vi "Translation3d_ToTranslation2d.vi"(11 "In Translation3d":T2 {"Z" format="%14.3f"; "Y" format="%14.3f"; "X" format="%14.3f"}) -> (3 "Translation2d":T1 {"Y" format="%14.3f"; "X" format="%14.3f"})   [LabVIEW 2019, in "Trajectory_Library.lvlib"]
doc: "Returns the X and Ycomponents of the translation.\n\nParameters\n - IN Translation - This Translation data structure\n\nReturns:\n - X- The X component of the translation.\n - Y- The Y component of the translation."
uses:
  TRANSLATION3D.ctl
  Trajectory_Library.lvlib
  TRANSLATION2D.ctl
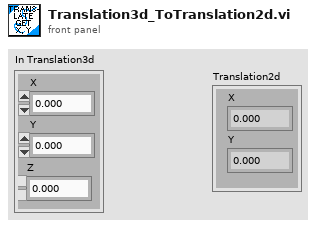
[diagram p1: front panel]
types:
  T1 = typedef "Trajectory_Library.lvlib/TRANSLATION2D.ctl" = cluster{"X":dbl, "Y":dbl}
  T2 = typedef "Trajectory_Library.lvlib/TRANSLATION3D.ctl" = cluster{"X":dbl, "Y":dbl, "Z":dbl}
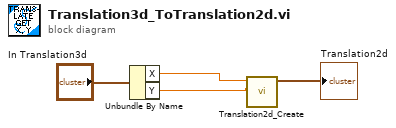
[diagram p0: block diagram]
diagram:
  n1 = Unbundle By Name("In Translation3d") -> ("X"=w2:dbl, "Y"=w1:dbl)
  n2 = call "Translation2d_Create.vi"("Y"=w1, "X"=w2) -> ("TRANSLATION"=→"Translation2d":T1)  [unwired: 9 in]
